vi "界面UI.vi"() -> ()   [LabVIEW 2016, in "科盛超标留样.lvlib"]
uses:
  <vilib>/Utility/miscctls.llb/LVPointTypeDef.ctl
  <vilib>/Utility/config.llb/NI_LVConfig.lvlib
panel:
  in  "返回":bool
  in  "查看记录":bool
  in  "当前解析模式":string(combo)
  in  "切换串口":bool
  out "查询系统状态":T1
  out "查询瓶记录":T2
  out "输出数组":T3(array[cluster])
  in  "留样命令":bool
  in  "供样命令":bool
  in  "触发采样":bool
  in  "查询系统状态":bool
  in  "远程取样":bool
  in  "复位指令":bool
  in  "查询瓶记录":bool
  in  "查询采样记录":bool
  in  "VISA resource name":refnum<visa-resource-name>="COM2" caption="VISA资源名称"
  in  "写入缓冲区":string
  out "读取缓冲区":string
  out "source":string
  out "通讯":bool
  # "科盛超标留样"
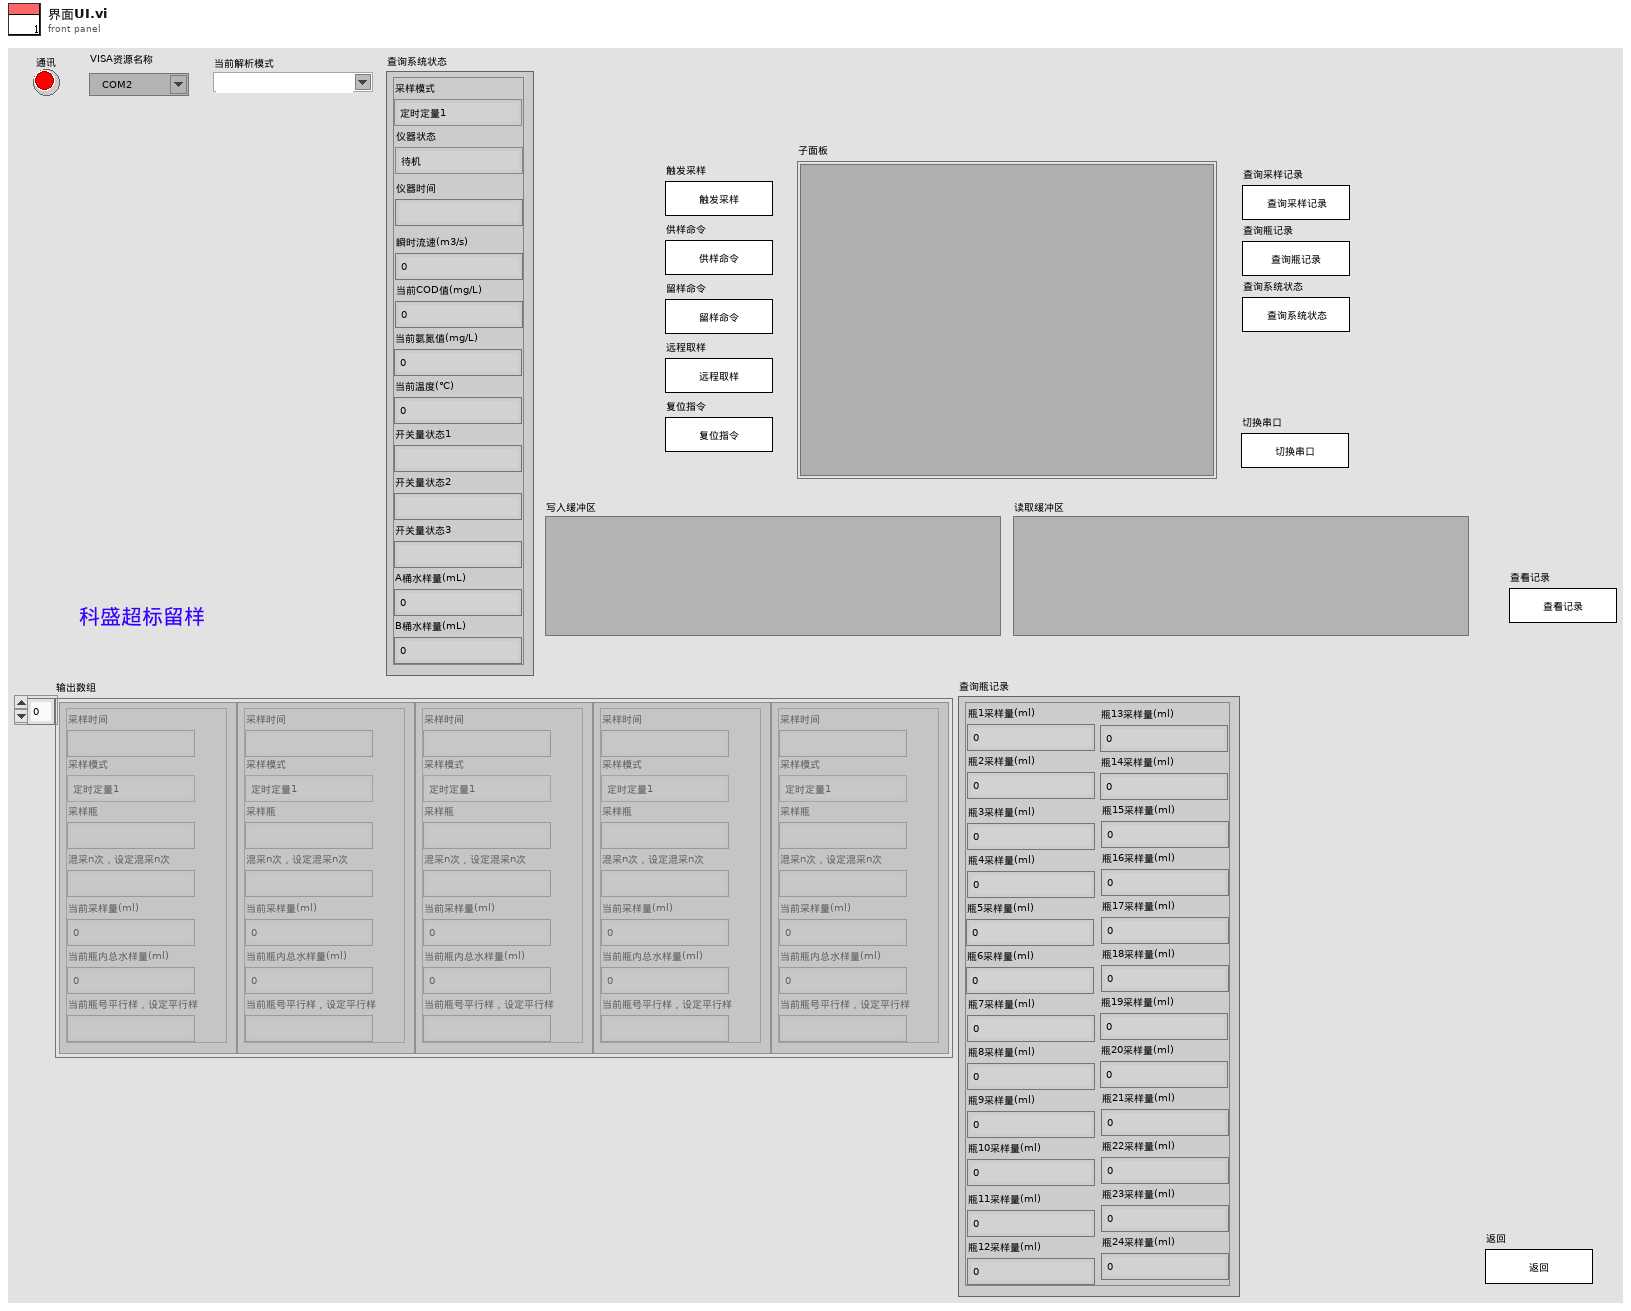
[diagram p1: front panel]
types:
  T1 = cluster{"采样模式":enum16{"定时定量1", "定时定量2", "定流定量", "定时比例", "同步留样", "超标留样", "触发采样", "定时采样1", "定流供样", "定时采样2", "远程取样", "手动取样", "流量跟踪"}, "仪器状态":enum16{"待机", "运行中"}, "仪器时间":string, "瞬时流速(m3/s)":dbl, "当前COD值(mg/L)":dbl, "当前氨氮值(mg/L)":dbl, "当前温度(℃)":dbl, "开关量状态1":string, "开关量状态2":string, "开关量状态3":string, "A桶水样量(mL)":dbl, "B桶水样量(mL)":dbl}
  T2 = cluster{"瓶1采样量(ml)":dbl, "瓶2采样量(ml)":dbl, "瓶3采样量(ml)":dbl, "瓶4采样量(ml)":dbl, "瓶5采样量(ml)":dbl, "瓶6采样量(ml)":dbl, "瓶7采样量(ml)":dbl, "瓶8采样量(ml)":dbl, "瓶9采样量(ml)":dbl, "瓶10采样量(ml)":dbl, "瓶11采样量(ml)":dbl, "瓶12采样量(ml)":dbl, "瓶13采样量(ml)":dbl, "瓶14采样量(ml)":dbl, "瓶15采样量(ml)":dbl, "瓶16采样量(ml)":dbl, "瓶17采样量(ml)":dbl, "瓶18采样量(ml)":dbl, "瓶19采样量(ml)":dbl, "瓶20采样量(ml)":dbl, "瓶21采样量(ml)":dbl, "瓶22采样量(ml)":dbl, "瓶23采样量(ml)":dbl, "瓶24采样量(ml)":dbl}
  T3 = cluster{"采样时间":string, "采样模式":enum16{"定时定量1", "定时定量2", "定流定量", "定时比例", "同步留样", "超标留样", "触发采样", "定时采样1", "定流供样", "定时采样2", "远程取样", "手动取样", "流量跟踪"}, "采样瓶":string, "混采n次，设定混采n次":string, "当前采样量(ml)":dbl, "当前瓶内总水样量(ml)":dbl, "当前瓶号平行样，设定平行样":string}[]
  T4 = cluster{"STEP":enum16{"open", "read", "write", "close"}, "写入缓冲区":string}
  T5 = enum16{"触发采样", "供样命令", "留样命令", "远程取样", "复位指令", "查询采样记录", "查询瓶记录", "查询系统状态"}
  T6 = typedef "LVPointTypeDef.ctl" = cluster{"Horizontal":i16, "Vertical":i16}
  T7 = typedef "NI_LVConfig.lvlib/Config Data RefNum.ctl" = refnum<k1>
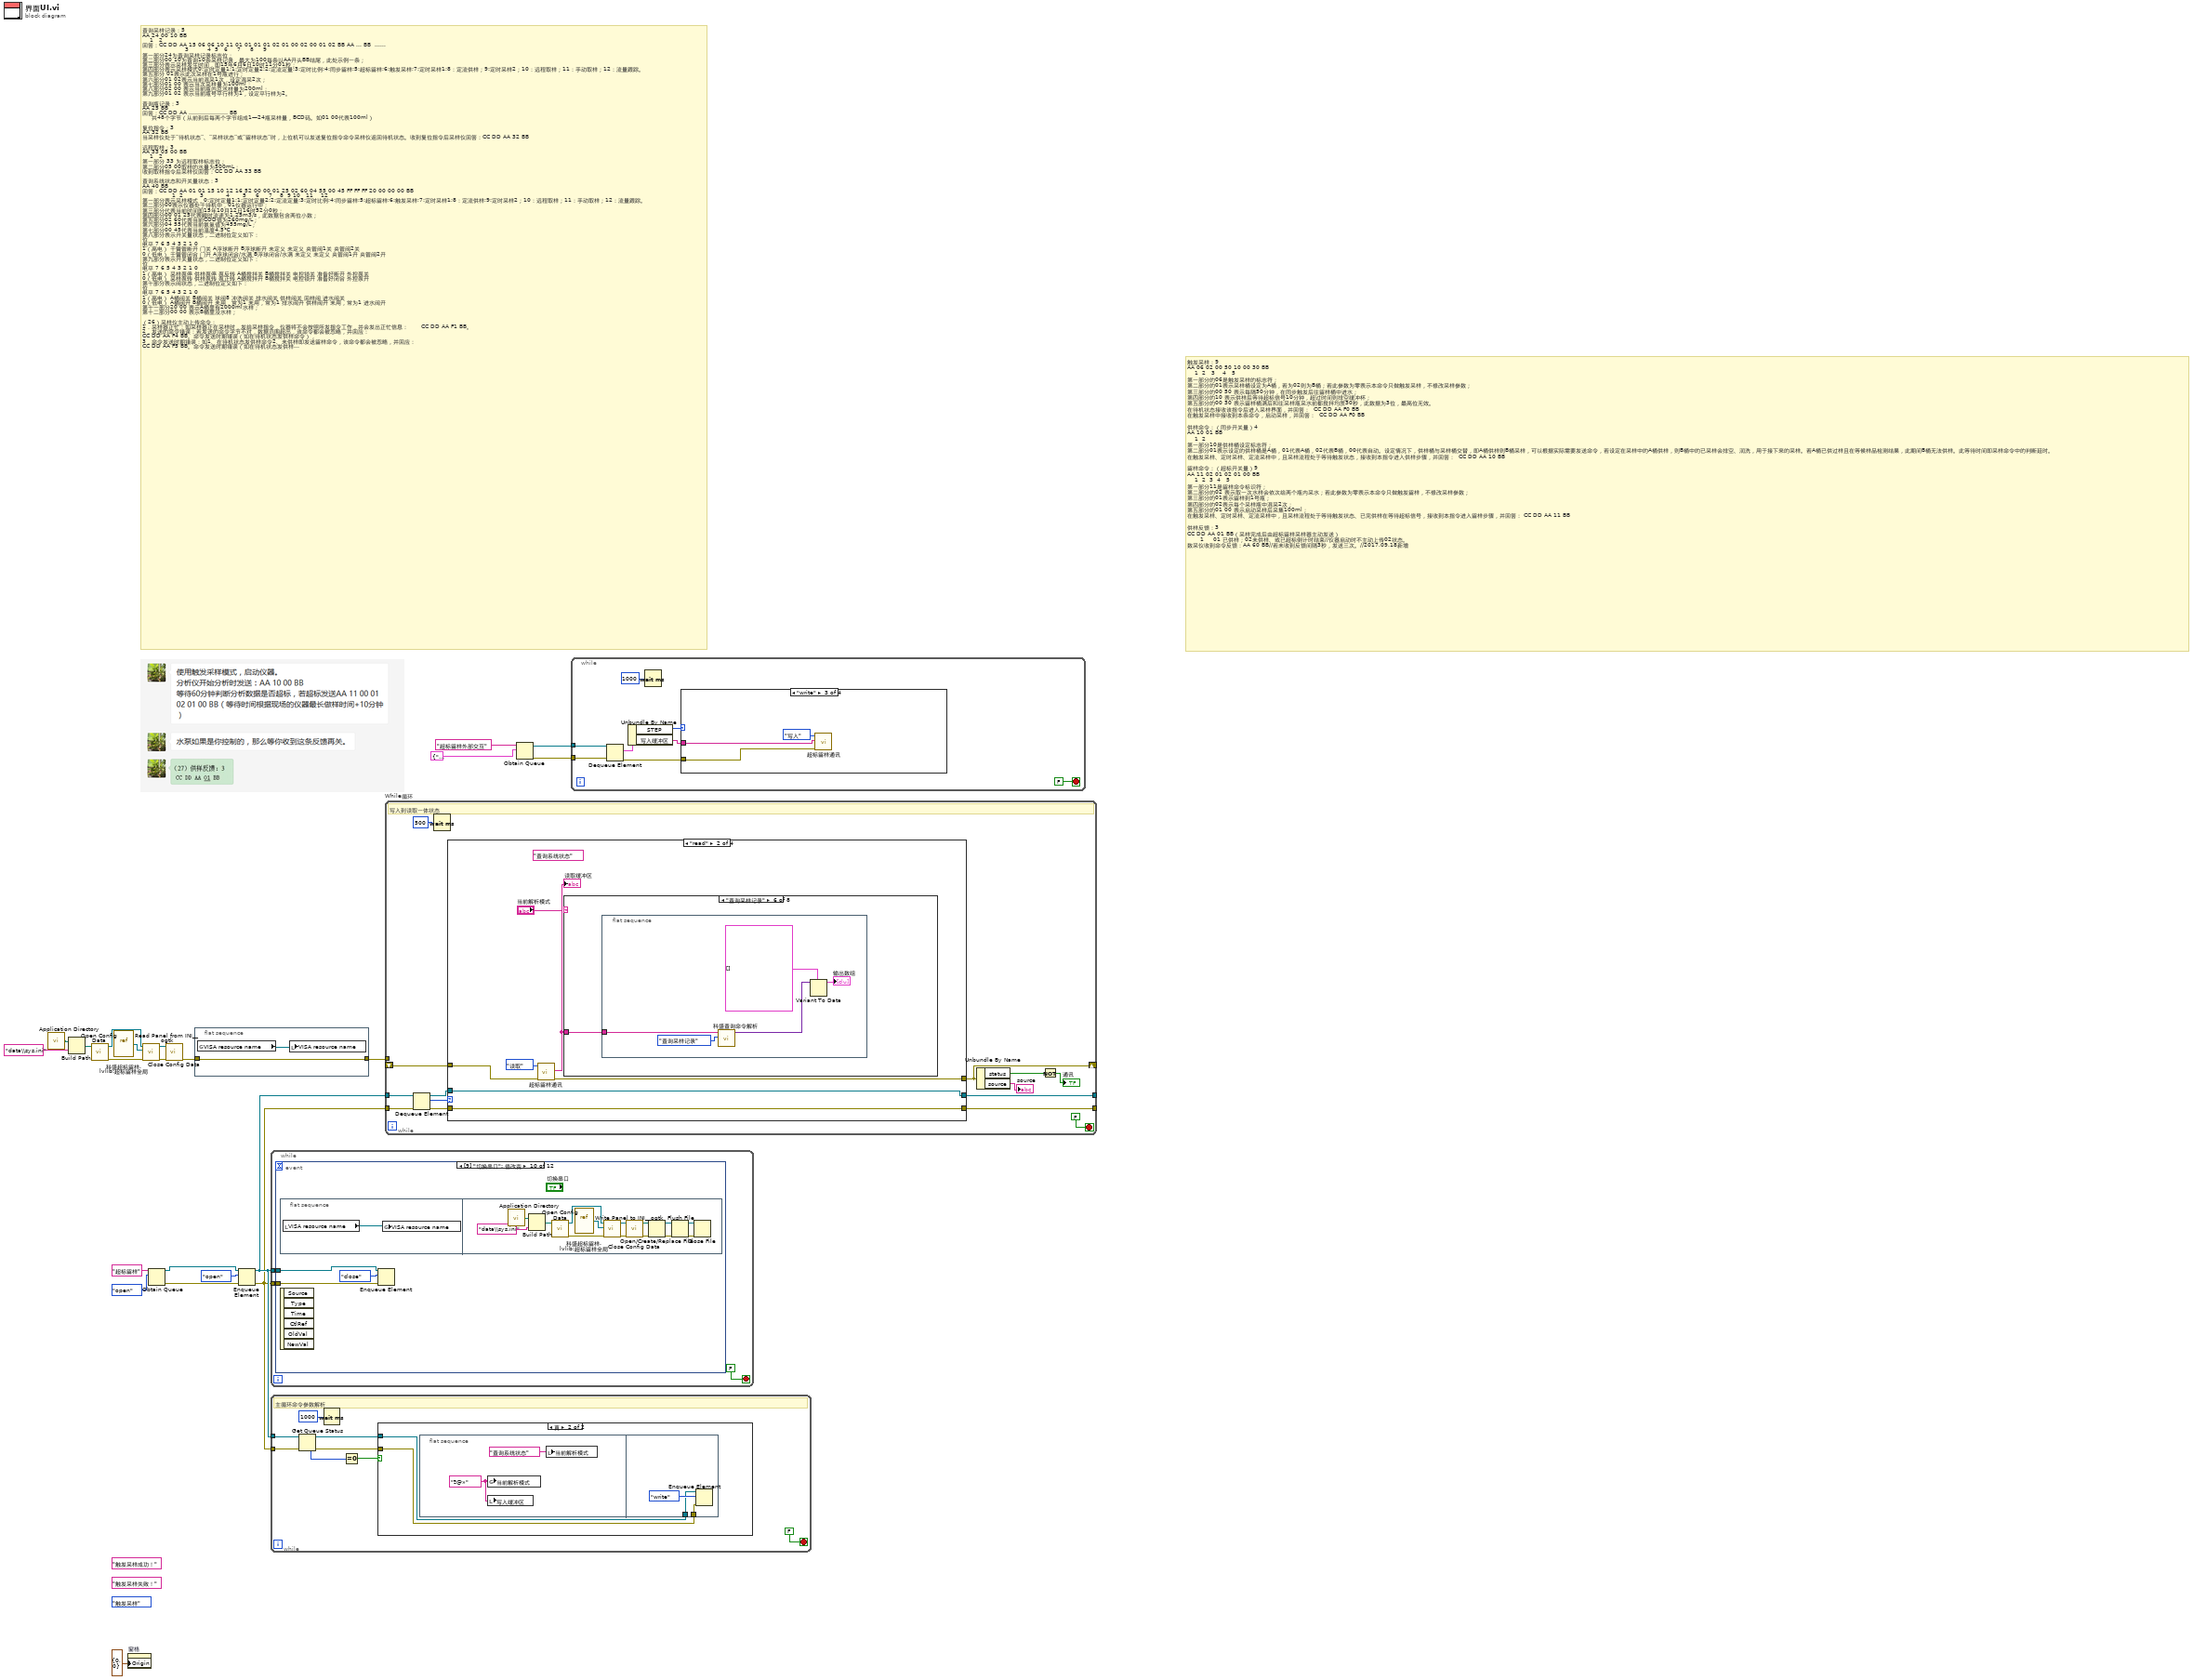
[diagram p0: block diagram]
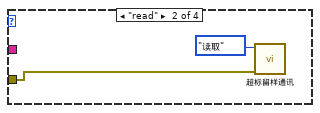
[diagram p3: hidden frame]
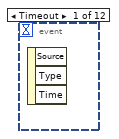
[diagram p6: hidden frame]
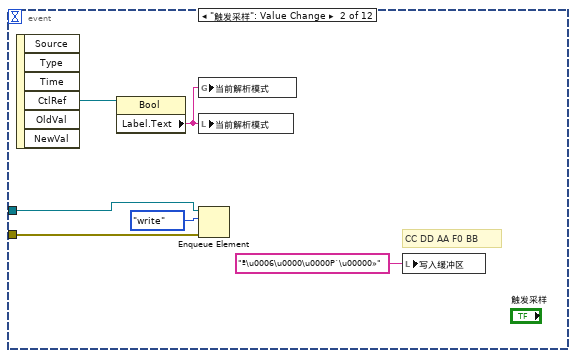
[diagram p7: hidden frame]
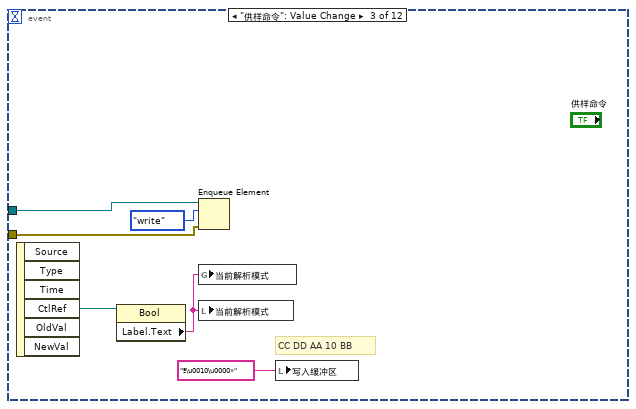
[diagram p8: hidden frame]
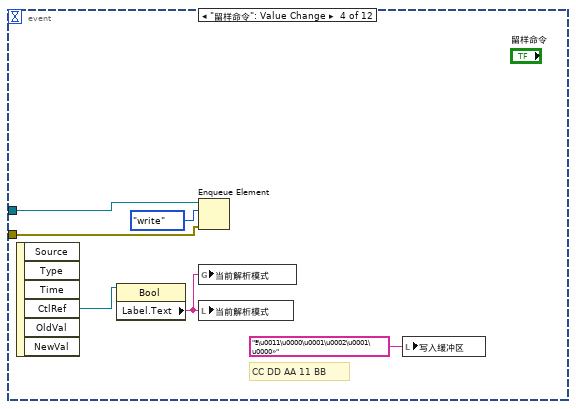
[diagram p9: hidden frame]
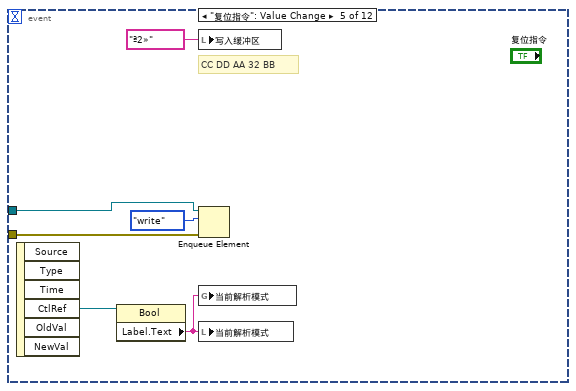
[diagram p10: hidden frame]
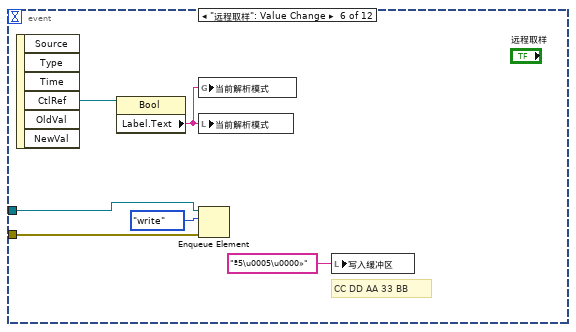
[diagram p11: hidden frame]
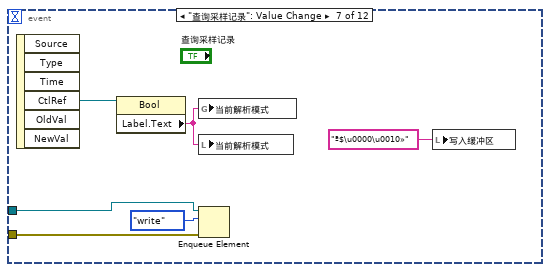
[diagram p12: hidden frame]
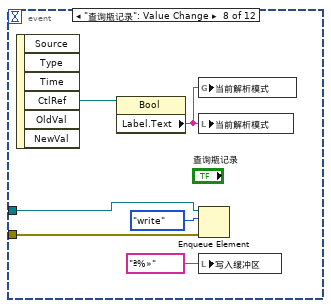
[diagram p13: hidden frame]
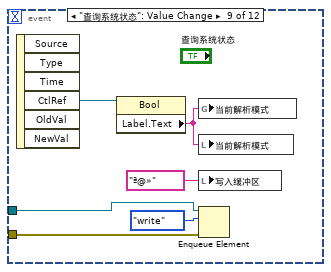
[diagram p14: hidden frame]
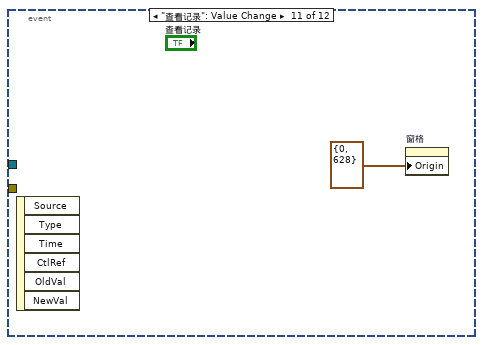
[diagram p15: hidden frame]
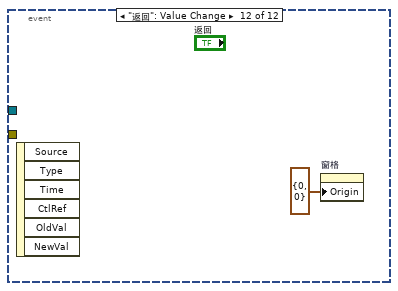
[diagram p16: hidden frame]
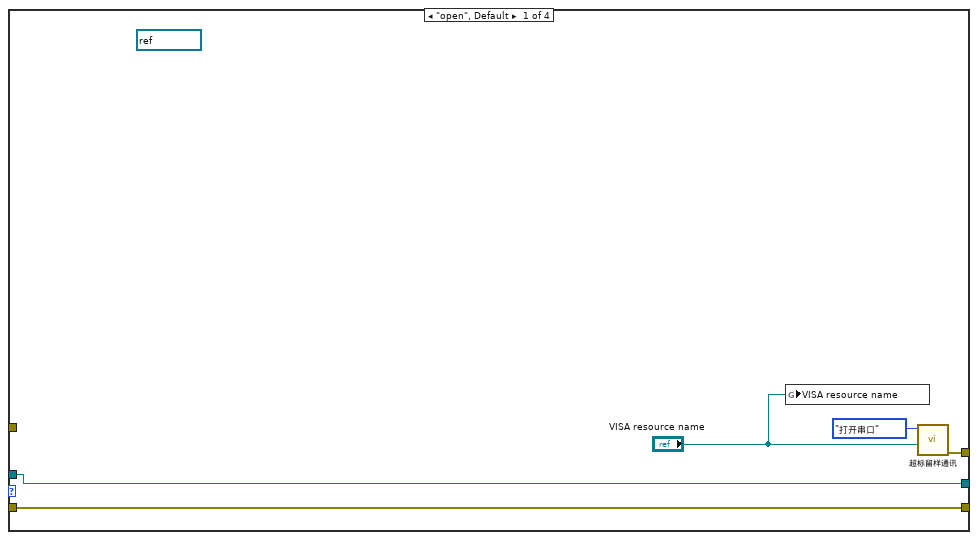
[diagram p17: hidden frame]
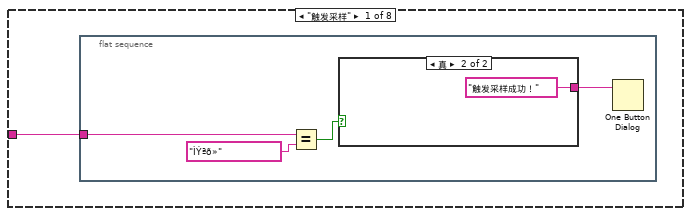
[diagram p18: hidden frame]
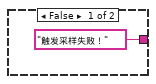
[diagram p19: hidden frame]
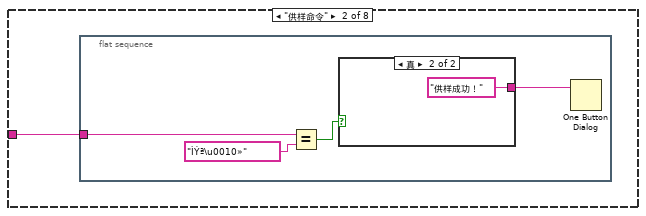
[diagram p20: hidden frame]
diagram:
  (unwired) "触发采样成功！" ("消息")
  (unwired) "触发采样失败！" ("消息")
  (unwired) T5."触发采样" ("功能输入")
  # "查询采样记录：5\nAA 24 00 10 BB\n    1   2\n回答：CC DD AA 15 06 06 10 11 01 01 01 01 02 01 00 02 00 01 02 BB AA ... BB  ......\n                       3          4  5   6     7     8     9\n第一部分24为查询采样记录标志位；\n第二部分00 10为查询10条采样记录，最大为100每条以AA开头BB结尾，此处示例一条；\n第三部分表示采样发生时间，即15年6月6日10时11分01秒；\n第四部分表示采样模式0:定时定量1;1:定时定量2;2:定流定量;3:定时比例;4:同步留样;5:超标留样;6:触发采样;7:定时采样1;8：定流供样；9:定时采样2；10：远程取样；11：手动取样；12：流量跟踪。\n第五部分 01表示此次采样在1号瓶进行；\n第六部分01 02表示当前混采1次，设定混采2次；\n第七部分01 00 表示当次采样量为100ml；\n第八部分02 00 表示当前瓶内总水样量为200ml；\n第九部分01 02 表示当前瓶号平行样为1，设定平行样为2。\n\n查询瓶记录：3\nAA 25 BB\n回答：CC DD AA ………………… BB\n     共48个字节（从前到后每两个字节组成1—24瓶采样量，BCD码。如01 00代表100ml）\n\n复位指令：3\nAA 32 BB\n当采样仪处于“待机状态”、“采样状态”或“留样状态”时，上位机可以发送复位指令命令采样仪返回待机状态。收到复位指令后采样仪回答：CC DD AA 32 BB\n\n远程取样：3\nAA 33 05 00 BB\n    1   2\n第一部分 33 为远程取样标志位；\n第二部分05 00取样的水量为500mL；\n收到取样指令后采样仪回答：CC DD AA 33 BB\n\n查询系统状态和开关量状态：3\nAA 40 BB\n回答：CC DD AA 01 01 15 10 12 16 52 00 00 01 25 02 60 04 55 00 45 FF FF FF 20 00 00 00 BB \n                1  2         3            4       5     6     7    8  9 10   11    12  \n第一部分表示采样模式，0:定时定量1;1:定时定量2;2:定流定量;3:定时比例;4:同步留样;5:超标留样;6:触发采样;7:定时采样1;8：定流供样;9:定时采样2；10：远程取样；11：手动取样；12：流量跟踪。\n第二部分00表示仪器处于待机中，01仪器运行中；\n第三部分代表当前时间即15年10月12日16时52分0秒； \n第四部分00 01 25代表瞬时流速为1.25m3/s，此数据包含两位小数；\n第五部分02 60代表当前COD值为260mg/L；\n第六部分04 55代表当前氨氮值为455mg/L；\n第七部分00 45代表当前温度4.5℃；\n第八部分表示开关量状态，二进制位定义如下：\n位\n电平\t7\t6\t5\t4\t3\t2\t1\t0\n1（高电）\t干簧管断开\t门关\tA浮球断开\tB浮球断开\t未定义\t未定义\t夹管阀1关\t夹管阀2关\n0（低电）\t干簧管闭合\t门开\tA浮球闭合/水满\tB浮球闭合/水满\t未定义\t未定义\t夹管阀1开\t夹管阀2开\n第九部分表示开关量状态，二进制位定义如下：\n位\n电平\t7\t6\t5\t4\t3\t2\t1\t0\n1（高电）\t采样泵停\t供样泵停\t泵反转\tA桶搅拌关\tB桶搅拌关\t电控锁关\t准备好断开\t外控泵关\n0（低电）\t采样泵转\t供样泵转\t泵正转\tA桶搅拌开\tB桶搅拌关\t电控锁开\t准备好闭合\t外控泵开\n第十部分表示阀状态，二进制位定义如下：\n位\n电平\t7\t6\t5\t4\t3\t2\t1\t0\n1（高电）\tA桶阀关\tB桶阀关\t球阀8\t冲洗阀关\t排水阀关\t供样阀关\t回样阀\t进水阀关\n0（低电）\tA桶阀开\tB桶阀开\t未用，常为1\t未用，常为1\t排水阀开\t供样阀开\t未用，常为1\t进水阀开\n第十一部分20 00 表示A桶里有2000ml水样；\n第十二部分00 00 表示B桶里没水样；\n\n（26）采样仪主动上传命令：\n1．采样器正忙：如采样器正在采样时，发给采样指令，仪器将不会按照所发指令工作，并会发出正忙信息：\t\t     CC DD AA F1 BB。\n2．发送的命令错误：若发送的命令字节不对，数据范围超出，该命令都会被忽略，并回应：\nCC DD AA F4 BB。命令发送时期错误（如在待机状态发供样命令），\n3．命令发送时期错误：如1、在待机状态发供样命令2、未供样即发送留样命令，该命令都会被忽略，并回应：\nCC DD AA F5 BB。命令发送时期错误（如在待机状态发供样命令），\n \t4．系统切换进入忙状态：仪器主动上传CC DD AA F6 BB。\n5．系统切换进入空闲状态：仪器主动上传CC DD AA F7 BB。"
  # "触发采样：9\nAA 06 02 00 50 10 00 30 BB\n    1  2   3    4   5         \n第一部分的06是触发采样的标志符；\n第二部分的01表示采样桶设定为A桶，若为02则为B桶；若此参数为零表示本命令只做触发采样，不修改采样参数；\n第三部分的00 50 表示每隔50分钟，在同步触发后往留样桶中进水；\n第四部分的10 表示供样后等待超标信号10分钟，超过时间则排空缓冲杯；\n第五部分的00 30 表示留样桶满后和往采样瓶采水前都搅拌均质30秒，此数据为3位，最高位无效。\n在待机状态接收该指令后进入采样界面，并回答：\t\tCC DD AA F0 BB\n在触发采样中接收到本条命令，启动采样，并回答：\t\tCC DD AA F0 BB\n\n供样命令：（同步开关量）4\nAA 10 01 BB\n    1  2  \n第一部分10是供样桶设定标志符；\n第二部分01表示设定的供样桶是A桶，01代表A桶，02代表B桶，00代表自动。设定情况下，供样桶与采样桶交替，即A桶供样则B桶采样，可以根据实际需要发送命令，若设定在采样中的A桶供样，则B桶中的已采样会排空、润洗，用于接下来的采样。若A桶已供过样且在等候样品检测结果，此期间B桶无法供样。此等待时间即采样命令中的判断延时。\n在触发采样、定时采样、定流采样中，且采样流程处于等待触发状态，接收到本指令进入供样步骤，并回答：\t\tCC DD AA 10 BB\n\n留样命令：（超标开关量）9\nAA 11 02 01 02 01 00 BB\n    1  2  3  4   5    \n第一部分11是留样命令标识符；\n第二部分的02 表示取一次水样会依次给两个瓶内采水；若此参数为零表示本命令只做触发留样，不修改采样参数；\n第三部分的01表示留样到1号瓶；\n第四部分的02表示每个采样瓶中混采2次；\n第五部分的01 00 表示启动采样后采集100ml；\n在触发采样、定时采样、定流采样中，且采样流程处于等待触发状态、已完供样在等待超标信号，接收到本指令进入留样步骤，并回答：\tCC DD AA 11 BB\n\n供样反馈：3\nCC DD AA 01 BB（采样完成后由超标留样采样器主动发送）\n  \t\t   1  \t\t\t01 已供样；02未供样、或已超标倒计时结束//仪器启动时不主动上传02状态。\n数采仪收到命令反馈：AA 60 BB//若未收到反馈间隔3秒，发送三次。//2017.09.18新增"
  n1 = call <vilib>:"Application Directory.vi"() -> ("Application Directory"=w14:path)
  n2 = Build Path(base path=w14, name or relative path="data\\sys.ini" ("名称或相对路径")) -> (appended path=w12:path)
  n3 = call <vilib>:"Open Config Data.vi"("configuration file path"=w12) -> ("error out"=w8:errorcluster, "refnum"=w11:T7)  [unwired: 8 in, 1 out]
  n4 = vi-ref "科盛超标留样.lvlib:超标留样全局.vi"() -> (w10:refnum<vi>)
  n5 = property on="窗格" class="Pane"("Origin"=T6 {"Horizontal"=0, "Vertical"=0} ("原点")) -> ()  [unwired: 2 in, 2 out]
  n6 = call <userlib>:"Read Panel from INI__ogtk.vi"("error in (no error)"=w8, "VI ref"=w10, "refnum"=w11) -> ("error out"=w7:errorcluster, "refnum out"=w9:T7)  [unwired: 7 in]
  n7 = Obtain Queue(name (unnamed)="超标留样" ("名称（未命名）"), element data type=enum16{"open", "read", "write", "close"}."open") -> (queue out=w20:refnum<queue>, error out=w19:errorcluster)  [unwired: 3 in, 1 out]
  n8 = call <vilib>:"Close Config Data.vi"("error in (no error)"=w7, "refnum"=w9) -> ("error out"=w6:errorcluster)  [unwired: 8 in, 1 out]
  n9 = flat-sequence {
    tunnel: w6 -> [w23]
    tunnel: [w23] -> w5
    frame #0 {
      n10 = global read "超标留样全局.vi" "VISA resource name"() -> (w24:refnum<visa-resource-name>)
      n11 = local write "VISA resource name"(w24) -> ()
    }
  }
  n12 = Enqueue Element(queue=w20, element=enum16{"open", "read", "write", "close"}."open", error in (no error)=w19) -> (queue out=w17:refnum<queue>, error out=w16:errorcluster)  [unwired: 1 in, 1 out]
  n13 = while {
    tunnel: w17 -> [w26]
    tunnel: w16 -> [w25]
    stop <- FALSE stop-if-true
    n14 = event shown="[9] \"切换串口\": 值改变" {
      selector: _ -> [_ _ _ _ _ _ _ _ _ _ _ _]
      dyn-events: _ -> [_ _ _ _ _ _ _ _ _ _ _ _]
      timeout: _ -> [_ _ _ _ _ _ _ _ _ _ _ _]
      tunnel: w26 -> [_ w32 w37 w44 w50 w56 w62 w68 w74 w76 _ _]
      tunnel: w25 -> [_ w31 w38 w43 w49 w55 w61 w67 w73 w77 _ _]
      event Timeout {
        n15 = event-data() -> ()  [unwired: 1 in, 3 out]
      }
      event "触发采样": Value Change {
        # "CC DD AA F0 BB"
        n16 = event-data() -> ("CtlRef"=w30:refnum<vi>)  [unwired: 1 in, 5 out]
        n17 = property class="Bool"(reference=w30) -> ("Label.Text"=w28:string)  [unwired: 1 in, 2 out]
        n18 = global write "超标留样全局.vi" "当前解析模式"(w28) -> ()
        n19 = local write "当前解析模式"(w28) -> ()
        n20 = Enqueue Element(queue=w32, element=enum16{"open", "read", "write", "close"}."write" ("元素"), error in (no error)=w31) -> ()  [unwired: 1 in, 3 out]
        n21 = local write "写入缓冲区"("ª\u0006\u0000\u0000P`\u00000»" ("写入缓冲区")) -> ()
      }
      event "供样命令": Value Change {
        # "CC DD AA 10 BB"
        n22 = event-data() -> ("CtlRef"=w36:refnum<vi>)  [unwired: 1 in, 5 out]
        n23 = property class="Bool"(reference=w36) -> ("Label.Text"=w34:string)  [unwired: 1 in, 2 out]
        n24 = Enqueue Element(queue=w37, element=enum16{"open", "read", "write", "close"}."write" ("元素"), error in (no error)=w38) -> ()  [unwired: 1 in, 3 out]
        n25 = global write "超标留样全局.vi" "当前解析模式"(w34) -> ()
        n26 = local write "当前解析模式"(w34) -> ()
        n27 = local write "写入缓冲区"("ª\u0010\u0000»" ("写入缓冲区")) -> ()
      }
      event "留样命令": Value Change {
        # "CC DD AA 11 BB"
        n28 = event-data() -> ("CtlRef"=w42:refnum<vi>)  [unwired: 1 in, 5 out]
        n29 = property class="Bool"(reference=w42) -> ("Label.Text"=w40:string)  [unwired: 1 in, 2 out]
        n30 = Enqueue Element(queue=w44, element=enum16{"open", "read", "write", "close"}."write" ("元素"), error in (no error)=w43) -> ()  [unwired: 1 in, 3 out]
        n31 = global write "超标留样全局.vi" "当前解析模式"(w40) -> ()
        n32 = local write "当前解析模式"(w40) -> ()
        n33 = local write "写入缓冲区"("ª\u0011\u0000\u0001\u0002\u0001\u0000»" ("写入缓冲区")) -> ()
      }
      event "复位指令": Value Change {
        # "CC DD AA 32 BB"
        n34 = event-data() -> ("CtlRef"=w48:refnum<vi>)  [unwired: 1 in, 5 out]
        n35 = property class="Bool"(reference=w48) -> ("Label.Text"=w46:string)  [unwired: 1 in, 2 out]
        n36 = local write "写入缓冲区"("ª2»" ("写入缓冲区")) -> ()
        n37 = Enqueue Element(queue=w50, element=enum16{"open", "read", "write", "close"}."write" ("元素"), error in (no error)=w49) -> ()  [unwired: 1 in, 3 out]
        n38 = global write "超标留样全局.vi" "当前解析模式"(w46) -> ()
        n39 = local write "当前解析模式"(w46) -> ()
      }
      event "远程取样": Value Change {
        # "CC DD AA 33 BB"
        n40 = event-data() -> ("CtlRef"=w54:refnum<vi>)  [unwired: 1 in, 5 out]
        n41 = property class="Bool"(reference=w54) -> ("Label.Text"=w52:string)  [unwired: 1 in, 2 out]
        n42 = global write "超标留样全局.vi" "当前解析模式"(w52) -> ()
        n43 = local write "当前解析模式"(w52) -> ()
        n44 = Enqueue Element(queue=w56, element=enum16{"open", "read", "write", "close"}."write" ("元素"), error in (no error)=w55) -> ()  [unwired: 1 in, 3 out]
        n45 = local write "写入缓冲区"("ª5\u0005\u0000»" ("写入缓冲区")) -> ()
      }
      event "查询采样记录": Value Change {
        n46 = event-data() -> ("CtlRef"=w60:refnum<vi>)  [unwired: 1 in, 5 out]
        n47 = property class="Bool"(reference=w60) -> ("Label.Text"=w58:string)  [unwired: 1 in, 2 out]
        n48 = global write "超标留样全局.vi" "当前解析模式"(w58) -> ()
        n49 = local write "当前解析模式"(w58) -> ()
        n50 = Enqueue Element(queue=w62, element=enum16{"open", "read", "write", "close"}."write" ("元素"), error in (no error)=w61) -> ()  [unwired: 1 in, 3 out]
        n51 = local write "写入缓冲区"("ª$\u0000\u0010»" ("写入缓冲区")) -> ()
      }
      event "查询瓶记录": Value Change {
        n52 = event-data() -> ("CtlRef"=w66:refnum<vi>)  [unwired: 1 in, 5 out]
        n53 = property class="Bool"(reference=w66) -> ("Label.Text"=w64:string)  [unwired: 1 in, 2 out]
        n54 = global write "超标留样全局.vi" "当前解析模式"(w64) -> ()
        n55 = local write "当前解析模式"(w64) -> ()
        n56 = Enqueue Element(queue=w68, element=enum16{"open", "read", "write", "close"}."write" ("元素"), error in (no error)=w67) -> ()  [unwired: 1 in, 3 out]
        n57 = local write "写入缓冲区"("ª%»" ("写入缓冲区")) -> ()
      }
      event "查询系统状态": Value Change {
        n58 = event-data() -> ("CtlRef"=w72:refnum<vi>)  [unwired: 1 in, 5 out]
        n59 = property class="Bool"(reference=w72) -> ("Label.Text"=w70:string)  [unwired: 1 in, 2 out]
        n60 = global write "超标留样全局.vi" "当前解析模式"(w70) -> ()
        n61 = local write "当前解析模式"(w70) -> ()
        n62 = local write "写入缓冲区"("ª@»" ("写入缓冲区")) -> ()
        n63 = Enqueue Element(queue=w74, element=enum16{"open", "read", "write", "close"}."write" ("元素"), error in (no error)=w73) -> ()  [unwired: 1 in, 3 out]
      }
      event "切换串口": Value Change {
        n64 = flat-sequence {
          frame #0 {
            n65 = local read "VISA resource name"() -> (w79:refnum<visa-resource-name>)
            n66 = global write "超标留样全局.vi" "VISA resource name"(w79) -> ()
          }
          frame #1 {
            n67 = call <vilib>:"Application Directory.vi"() -> ("Application Directory"=w81:path)
            n68 = Build Path(base path=w81, name or relative path="data\\sys.ini" ("名称或相对路径")) -> (appended path=w82:path)
            n69 = call <vilib>:"Open Config Data.vi"("configuration file path"=w82) -> ("error out"=w86:errorcluster, "refnum"=w83:T7)  [unwired: 8 in, 1 out]
            n70 = vi-ref "科盛超标留样.lvlib:超标留样全局.vi"() -> (w84:refnum<vi>)
            n71 = call <userlib>:"Write Panel to INI__ogtk.vi"("error in (no error)"=w86, "VI ref"=w84, "refnum"=w83) -> ("error out"=w87:errorcluster, "refnum out"=w85:T7)  [unwired: 7 in]
            n72 = call <vilib>:"Close Config Data.vi"("error in (no error)"=w87, "refnum"=w85) -> ("error out"=w92:errorcluster, "file path"=w93:path)  [unwired: 8 in]
            n73 = Open/Create/Replace File(file path (use dialog)=w93, error in=w92) -> (refnum out=w89:refnum<file>, error out=w88:errorcluster)  [unwired: 4 in, 1 out]
            n74 = Flush File(refnum=w89, error in=w88) -> (refnum out=w90:refnum<file>, error out=w91:errorcluster)
            n75 = Close File(refnum=w90, error in=w91) -> ()  [unwired: 2 out]
          }
        }
        n76 = event-data() -> ()  [unwired: 1 in, 6 out]
        n77 = Enqueue Element(queue=w76, element=enum16{"open", "read", "write", "close"}."close" ("元素"), error in (no error)=w77) -> ()  [unwired: 1 in, 3 out]
      }
      event "查看记录": Value Change {
        n78 = event-data() -> ()  [unwired: 1 in, 6 out]
        n79 = property on="窗格" class="Pane"("Origin"=T6 {"Horizontal"=0, "Vertical"=628} ("原点")) -> ()  [unwired: 2 in, 2 out]
      }
      event "返回": Value Change {
        n80 = event-data() -> ()  [unwired: 1 in, 6 out]
        n81 = property on="窗格" class="Pane"("Origin"=T6 {"Horizontal"=0, "Vertical"=0} ("原点")) -> ()  [unwired: 2 in, 2 out]
      }
    }
  }
  n82 = while {
    tunnel: w17 -> [w101]
    tunnel: w16 -> [w100]
    stop <- FALSE stop-if-true
    # "主循环命令参数解析"
    n83 = Get Queue Status(queue=w101, error in (no error)=w100) -> (queue out=w97:refnum<queue>, error out=w96:errorcluster, # elements in queue=w99:i32)  [unwired: 1 in, 5 out]
    n84 = Wait (ms)(milliseconds to wait=u32 1000 ("等待时间（毫秒）")) -> ()  [unwired: 1 out]
    n85 = Equal To 0?(x=w99) -> (x = 0?=w98:bool)
    n86 = case shown="真" w98 {
      tunnel: w97 -> [_ w105]
      tunnel: w96 -> [_ w104]
      frame False {
      }
      frame True {
        n87 = flat-sequence {
          tunnel: w105 -> [w109]
          tunnel: w104 -> [w108]
          frame #0 {
            w107 = "ª@»" ("写入缓冲区")
            n88 = global write "超标留样全局.vi" "当前解析模式"(w107) -> ()
            n89 = local write "写入缓冲区"(w107) -> ()
            n90 = local write "当前解析模式"("查询系统状态" ("当前解析模式")) -> ()
          }
          frame #1 {
            n91 = Enqueue Element(queue=w109, element=enum16{"open", "read", "write", "close"}."write" ("元素"), error in (no error)=w108) -> ()  [unwired: 1 in, 3 out]
          }
        }
      }
    }
  }
  n92 = while "While循环" {
    tunnel: w17 -> [w122]
    tunnel: w16 -> [w121]
    tunnel: [w117] -> _
    tunnel: [w116] -> _
    shift-right: [w111] -> _
    shift-left: _ -> [w115]
    tunnel: w5 -> [_]
    stop <- FALSE stop-if-true
    # "写入到读取一体状态"
    n93 = Dequeue Element(queue=w122, error in (no error)=w121) -> (queue out=w119:refnum<queue>, element=w120:enum16{"open", "read", "write", "close"}, error out=w118:errorcluster)  [unwired: 1 in, 1 out]
    n94 = Wait (ms)(milliseconds to wait=u32 500 ("等待时间（毫秒）")) -> ()  [unwired: 1 out]
    n95 = case shown="\"read\"" w120 {
      tunnel: [w128 w135 w193 w205] -> w111
      tunnel: w119 -> [w127 w133 w198 w204]
      tunnel: w118 -> [w126 w132 w197 w203]
      tunnel: [w127 w133 w196 w201] -> w117
      tunnel: [w126 w132 w195 w200] -> w116
      tunnel: w115 -> [_ w136 w194 w207]
      frame "open", Default {
        (unwired) refnum<visa-resource-name> "COM2" ("VISA resource name")
        n96 = global write "超标留样全局.vi" "VISA resource name"("VISA resource name") -> ()
        n97 = call "超标留样通讯.vi"("VISA resource name"="VISA resource name", "功能输入"=enum16{"打开串口", "写入", "读取", "关闭串口"}."打开串口") -> ("error out"=w128:errorcluster)  [unwired: 7 in, 2 out]
      }
      frame "read" {
        (unwired) "查询系统状态" ("当前解析模式")
        n98 = call "超标留样通讯.vi"("error in (no error)"=w136, "功能输入"=enum16{"打开串口", "写入", "读取", "关闭串口"}."读取") -> ("error out"=w135:errorcluster, "读取缓冲区"=w131:string)  [unwired: 7 in, 1 out]
        "读取缓冲区" <- w131
        n99 = case shown="\"查询采样记录\"" "当前解析模式" {
          tunnel: w131 -> [w137 w144 w151 w158 w165 w172 w178 w184]
          frame "触发采样" {
            n100 = flat-sequence {
              tunnel: w137 -> [w141]
              frame #0 {
                n101 = Equal?(x=w141, y="ÌÝªð»") -> (x = y?=w139:bool)
                n102 = case shown="真" w139 {
                  tunnel: ["触发采样失败！" ("消息") "触发采样成功！" ("消息")] -> w138
                  frame False {
                  }
                  frame True {
                  }
                }
                n103 = One Button Dialog(message=w138) -> ()  [unwired: 1 in, 1 out]
              }
            }
          }
          frame "供样命令" {
            n104 = flat-sequence {
              tunnel: w144 -> [w148]
              frame #0 {
                n105 = Equal?(x=w148, y="ÌÝª\u0010»") -> (x = y?=w146:bool)
                n106 = case shown="真" w146 {
                  tunnel: ["供样失败！" ("消息") "供样成功！" ("消息")] -> w145
                  frame False {
                  }
                  frame True {
                  }
                }
                n107 = One Button Dialog(message=w145) -> ()  [unwired: 1 in, 1 out]
              }
            }
          }
          frame "留样命令", Default {
            n108 = flat-sequence {
              tunnel: w151 -> [w155]
              frame #0 {
                n109 = Equal?(x=w155, y="ÌÝª\u0011»") -> (x = y?=w153:bool)
                n110 = case shown="真" w153 {
                  tunnel: ["留样失败！" ("消息") "留样成功！" ("消息")] -> w152
                  frame False {
                  }
                  frame True {
                  }
                }
                n111 = One Button Dialog(message=w152) -> ()  [unwired: 1 in, 1 out]
              }
            }
          }
          frame "复位指令" {
            n112 = flat-sequence {
              tunnel: w158 -> [w162]
              frame #0 {
                n113 = Equal?(x=w162, y="ÌÝª2»") -> (x = y?=w160:bool)
                n114 = case shown="真" w160 {
                  tunnel: ["复位失败！" ("消息") "复位成功！" ("消息")] -> w159
                  frame False {
                  }
                  frame True {
                  }
                }
                n115 = One Button Dialog(message=w159) -> ()  [unwired: 1 in, 1 out]
              }
            }
          }
          frame "远程取样" {
            n116 = flat-sequence {
              tunnel: w165 -> [w169]
              frame #0 {
                n117 = Equal?(x=w169, y="ÌÝª3»") -> (x = y?=w167:bool)
                n118 = case shown="假" w167 {
                  tunnel: ["远程取样失败！" ("消息") "远程取样成功！" ("消息")] -> w166
                  frame False {
                  }
                  frame True {
                  }
                }
                n119 = One Button Dialog(message=w166) -> ()  [unwired: 1 in, 1 out]
              }
            }
          }
          frame "查询采样记录" {
            n120 = flat-sequence {
              tunnel: w172 -> [w177]
              frame #0 {
                n121 = call "科盛查询命令解析.vi"("解析参数选择"=enum16{"查询采样记录", "查询瓶记录", "查询系统状态"}."查询采样记录", "命令输入"=w177) -> ("Variant"=w175:variant)  [unwired: 9 in]
                n122 = Variant To Data(type=T3 [] ("输出数组"), Variant=w175) -> (data=→"输出数组":T3)  [unwired: 1 in, 1 out]
              }
            }
          }
          frame "查询瓶记录" {
            n123 = flat-sequence {
              tunnel: w178 -> [w183]
              frame #0 {
                n124 = call "科盛查询命令解析.vi"("解析参数选择"=enum16{"查询采样记录", "查询瓶记录", "查询系统状态"}."查询瓶记录", "命令输入"=w183) -> ("Variant"=w181:variant)  [unwired: 9 in]
                n125 = Variant To Data(type=T2 {"瓶1采样量(ml)"=0.0, "瓶2采样量(ml)"=0.0, "瓶3采样量(ml)"=0.0, "瓶4采样量(ml)"=0.0, "瓶5采样量(ml)"=0.0, "瓶6采样量(ml)"=0.0, "瓶7采样量(ml)"=0.0, "瓶8采样量(ml)"=0.0, "瓶9采样量(ml)"=0.0, "瓶10采样量(ml)"=0.0, "瓶11采样量(ml)"=0.0, "瓶12采样量(ml)"=0.0, "瓶13采样量(ml)"=0.0, "瓶14采样量(ml)"=0.0, "瓶15采样量(ml)"=0.0, "瓶16采样量(ml)"=0.0, "瓶17采样量(ml)"=0.0, "瓶18采样量(ml)"=0.0, "瓶19采样量(ml)"=0.0, "瓶20采样量(ml)"=0.0, "瓶21采样量(ml)"=0.0, "瓶22采样量(ml)"=0.0, "瓶23采样量(ml)"=0.0, "瓶24采样量(ml)"=0.0} ("查询瓶记录"), Variant=w181) -> (data=→"查询瓶记录":T2)  [unwired: 1 in, 1 out]
              }
            }
          }
          frame "查询系统状态" {
            n126 = flat-sequence {
              tunnel: w184 -> [w189]
              frame #0 {
                n127 = call "科盛查询命令解析.vi"("解析参数选择"=enum16{"查询采样记录", "查询瓶记录", "查询系统状态"}."查询系统状态", "命令输入"=w189) -> ("Variant"=w187:variant)  [unwired: 9 in]
                n128 = Variant To Data(type=T1 {"采样模式"=enum."定时定量1", "仪器状态"=enum."待机", "仪器时间"="", "瞬时流速(m3/s)"=0.0, "当前COD值(mg/L)"=0.0, "当前氨氮值(mg/L)"=0.0, "当前温度(℃)"=0.0, "开关量状态1"="", "开关量状态2"="", "开关量状态3"="", "A桶水样量(mL)"=0.0, "B桶水样量(mL)"=0.0} ("查询系统状态"), Variant=w187) -> (data=→"查询系统状态":T1)  [unwired: 1 in, 1 out]
              }
            }
          }
        }
      }
      frame "write" {
        n129 = Wait (ms)(milliseconds to wait=u32 500 ("等待时间（毫秒）")) -> ()  [unwired: 1 out]
        n130 = Enqueue Element(queue=w198, element=enum16{"open", "read", "write", "close"}."read" ("元素"), error in (no error)=w197) -> (queue out=w196:refnum<queue>, error out=w195:errorcluster)  [unwired: 1 in, 1 out]
        n131 = call "超标留样通讯.vi"("error in (no error)"=w194, "写入缓冲区"="写入缓冲区", "功能输入"=enum16{"打开串口", "写入", "读取", "关闭串口"}."写入") -> ("error out"=w193:errorcluster)  [unwired: 6 in, 2 out]
      }
      frame "close" {
        n132 = Enqueue Element(queue=w204, element=enum16{"open", "read", "write", "close"}."open" ("元素"), error in (no error)=w203) -> (queue out=w201:refnum<queue>, error out=w200:errorcluster)  [unwired: 1 in, 1 out]
        n133 = call "超标留样通讯.vi"("error in (no error)"=w207, "功能输入"=enum16{"打开串口", "写入", "读取", "关闭串口"}."关闭串口") -> ("error out"=w205:errorcluster)  [unwired: 7 in, 2 out]
      }
    }
    n134 = Unbundle By Name(w111) -> ("status"=w113:bool, "source"=→"source":string)
    n135 = Not(x=w113) -> (.not. x?=→"通讯":bool)
  }
  n136 = Obtain Queue(name (unnamed)="超标留样外部交互" ("名称（未命名）"), element data type=T4 {"STEP"=enum."write", "写入缓冲区"="ª\u0006\u0000\u0000P`\u00000»"}) -> (queue out=w2:refnum<queue>, error out=w1:errorcluster)  [unwired: 3 in, 1 out]
  n137 = while {
    tunnel: w2 -> [w213]
    tunnel: w1 -> [w212]
    stop <- FALSE stop-if-true
    n138 = Dequeue Element(queue=w213, error in (no error)=w212) -> (element=w211:T4, error out=w209:errorcluster)  [unwired: 1 in, 2 out]
    n139 = Unbundle By Name(w211) -> ("STEP"=w210:enum16{"open", "read", "write", "close"}, "写入缓冲区"=w208:string)
    n140 = Wait (ms)(milliseconds to wait=u32 1000 ("等待时间（毫秒）")) -> ()  [unwired: 1 out]
    n141 = case shown="\"write\"" w210 {
      tunnel: w209 -> [_ w216 w219 _]
      tunnel: w208 -> [_ _ w218 _]
      frame "open", Default {
      }
      frame "read" {
        n142 = call "超标留样通讯.vi"("error in (no error)"=w216, "功能输入"=enum16{"打开串口", "写入", "读取", "关闭串口"}."读取") -> ()  [unwired: 7 in, 3 out]
      }
      frame "write" {
        n143 = call "超标留样通讯.vi"("error in (no error)"=w219, "写入缓冲区"=w218, "功能输入"=enum16{"打开串口", "写入", "读取", "关闭串口"}."写入") -> ()  [unwired: 6 in, 3 out]
      }
      frame "close" {
      }
    }
  }
